vi "Get.vi"(6 "Pretty print":bool=TRUE, 8 "error in":errorcluster, 9 "Filtering Params":T1[](array[typedef]), 10 "endPoint":string, 11 "firebase in":refnum<class "firebase.lvclass">) -> (0 "error out":errorcluster, 2 "Json String":string, 3 "firebase out":refnum<class "firebase.lvclass">)   [LabVIEW 2019, in "firebase.lvclass"]
uses:
  firebase.lvclass
  Filtering Parameters--cluster.ctl
  <vilib>/JDP Science/JSONtext/Next JSON Value.vi
  <vilib>/JDP Science/JSONtext/String Subset.vi
  <vilib>/JDP Science/JSONtext/Parsing/Advance past next JSON Value (inlined COPY).vi
  <vilib>/JDP Science/JSONtext/Parsing/Advance past whitespace.vi
  <vilib>/JDP Science/JSONtext/Parsing/Advance past String.vi
  <vilib>/JDP Science/JSONtext/Parsing/Advance past Number.vi
  <vilib>/JDP Science/JSONtext/Parsing/Advance past Line Ending.vi
  <vilib>/JDP Science/JSONtext/Parsing/Parse Full Path or Item Name.vi
  <vilib>/JDP Science/JSONtext/Parsing/Advance past Array.vi
  <vilib>/JDP Science/JSONtext/Parsing/Advance past Object.vi
  <vilib>/JDP Science/JSONtext/support/Error Cluster From Code.vi
  <vilib>/JDP Science/JSONtext/Offset/Find Item Locations by Path.vi
  <vilib>/JDP Science/JSONtext/JSON text to Variant.vi
  <vilib>/JDP Science/JSONtext/LVClass Serializer/JSONtext LVClass Serializer.lvclass
  <vilib>/NI/Advanced HTTP Client/Session.lvclass
  <vilib>/JDP Science/JSONtext/JSONtext.lvlib
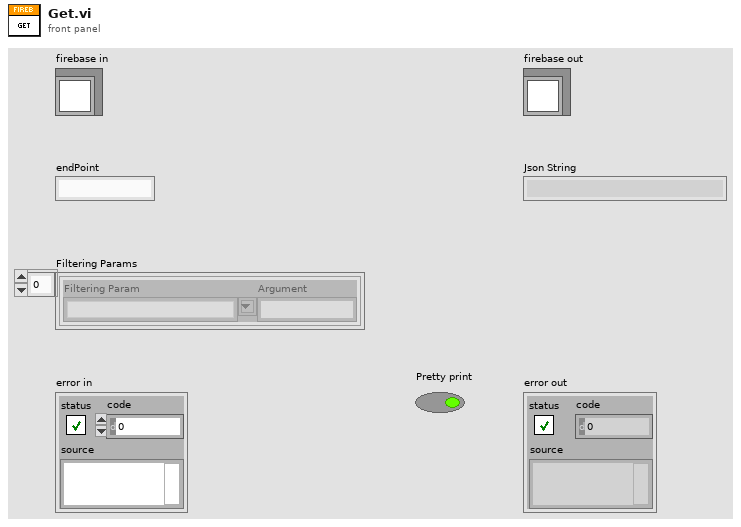
[diagram p1: front panel]
types:
  T1 = typedef "firebase.lvclass/Filtering Parameters--cluster.ctl" = cluster{"Filtering Param":string, "Argument":string}
  T2 = typedef "firebase.lvclass/Success Sign In--cluster.ctl" = cluster{"kind":string, "idToken":string, "email":string, "refreshToken":string, "expiresIn":string, "localId":string, "displayName":string, "registered":bool}
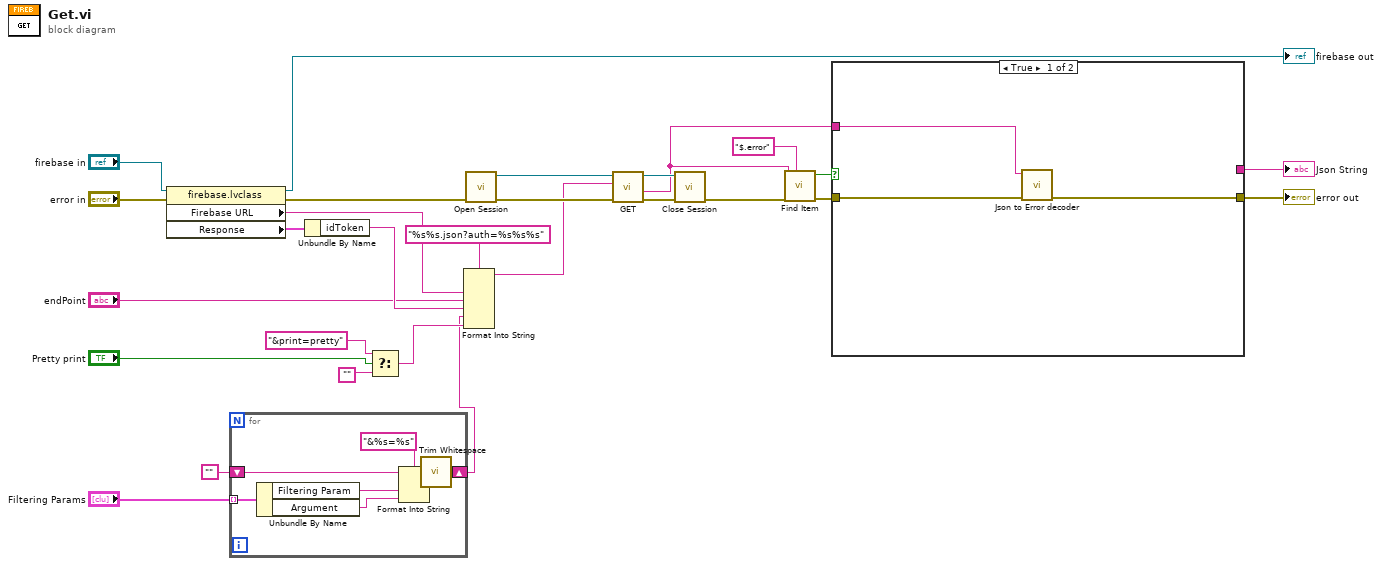
[diagram p0: block diagram]
diagram:
  n1 = property class="firebase.lvclass"(reference="firebase in", error in="error in") -> (reference out=→"firebase out":refnum<class "firebase.lvclass">, error out=w24:errorcluster, "Firebase URL"=w19:string, "Response"=w11:T2)
  n2 = for {
    tunnel: "Filtering Params" -> [w35] mode=indexing
    shift-right: [w29] -> w1
    shift-left: "" -> [w30]
    n3 = Unbundle By Name(w35) -> ("Filtering Param"=w34:string, "Argument"=w33:string)
    n4 = Format Into String(format string="&%s=%s", initial string=w30, w34, w33) -> (resulting string=w32:string)  [unwired: 1 in, 1 out]
    n5 = call <vilib>:"Trim Whitespace.vi"("string"=w32) -> ("trimmed string"=w29:string)  [unwired: 1 in]
  }
  n6 = Unbundle By Name(w11) -> ("idToken"=w10:string)
  n7 = Select(t="&print=pretty" ("format string"), s="Pretty print", f="") -> (s? t:f=w2:string)
  n8 = Format Into String(format string="%s%s.json?auth=%s%s%s", w19, "endPoint", w10, w1, w2) -> (resulting string=w15:string)  [unwired: 2 in, 1 out]
  n9 = call <vilib>:"Open Session.vi"("error in"=w24) -> ("error out"=w26:errorcluster, "session"=w16:refnum<class "Session.lvclass">)  [unwired: 9 in]
  n10 = call <vilib>:"GET.vi"("error in"=w26, "url"=w15, "session in"=w16) -> ("error out"=w27:errorcluster, "body"=w12:string, "session out"=w17:refnum<class "Session.lvclass">)  [unwired: 4 in, 2 out]
  n11 = call <vilib>:"Close Session.vi"("error in"=w27, "session"=w17) -> ("error out"=w23:errorcluster)  [unwired: 9 in]
  n12 = call <vilib>:"Find Item.vi"("$Path or Item Name"="$.error", "error in (no error)"=w23, "JSON"=w12) -> ("error out"=w25:errorcluster, "Found"=w13:bool)  [unwired: 5 in, 2 out]
  n13 = case shown="True" w13 {
    tunnel: [w37 w40] -> w22
    tunnel: w25 -> [w38 w40]
    tunnel: w12 -> [w36 w39]
    tunnel: [_ w39] -> w8
    frame True {
      n14 = call "Json to Error decoder.vi"("error in"=w38, "body"=w36) -> ("error out"=w37:errorcluster)  [unwired: 9 in]
    }
    frame False {
    }
  }
  "error out" <- w22
  "Json String" <- w8
